vi "start_photon_stream.vi"(8 "error in (no error)":errorcluster, 11 "tt20 in":refnum<class "tt20.lvclass">) -> (0 "error out":errorcluster, 3 "tt20 out":refnum<class "tt20.lvclass">)   [LabVIEW 2015, in "tt20.lvclass"]
uses:
  tt20.lvclass
  tt20.lvclass/tt20.ctl
  tt20_buffer_tdef.ctl
  C:/Users/MX-Microscope/Documents/LabVIEW Data/lvoop_campus_2018/Detector_Class/Swabian/time_tagger_vis/TTCSharp32.dll
  time_tagger_vis/TTCSharp32.dll
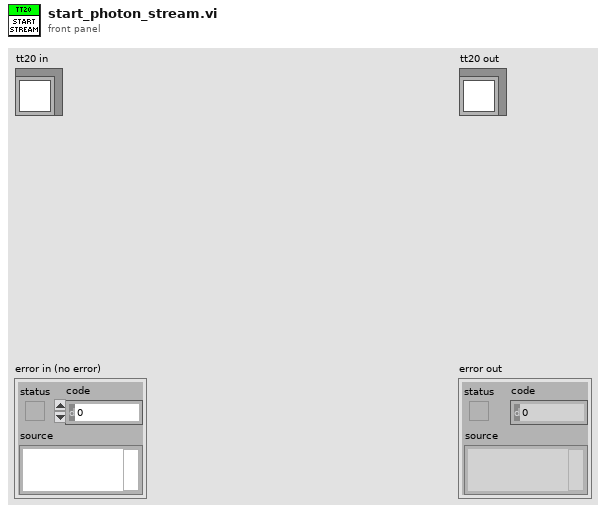
[diagram p1: front panel]
types:
  T1 = typedef "tt20_buffer_tdef.ctl" = cluster{"tagChannels":u32[], "tagTimestamps":i64[], "size":i32}
  T2 = typedef "tt20_acq_mode_tdef.ctl" = enum16{"T2", "T3"}
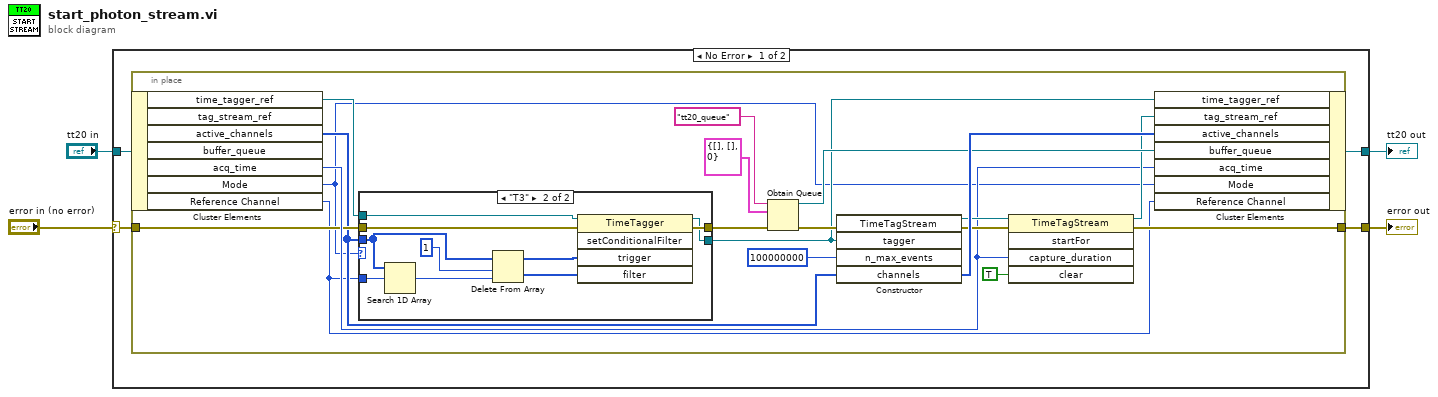
[diagram p0: block diagram]
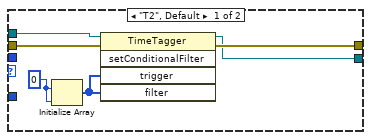
[diagram p2: hidden frame]
diagram:
  n1 = case shown="No Error" "error in (no error)" {
    selector: "error in (no error)" -> [w7 w44]
    tunnel: "tt20 in" -> [w8 w45]
    tunnel: [w6 w44] -> w2
    tunnel: [w5 w45] -> w1
    frame No Error {
      n2 = in-place {
        in-place-border: w7 -> [w15]
        in-place-border: [w19] -> w6
        n3 = in-place-cluster #1(w8) -> ("time_tagger_ref"=w13:refnum<k24>, "active_channels"=w11:u32[], "acq_time"=w16:i64, "Mode"=w10:T2, "Reference Channel"=w9:u8)  [unwired: 2 out]
        n4 = case shown="\"T3\"" w10 {
          tunnel: w15 -> [w33 w43]
          tunnel: [w32 w42] -> w14
          tunnel: w13 -> [w31 w41]
          tunnel: [w30 w40] -> w12
          tunnel: w11 -> [_ w38]
          tunnel: w9 -> [_ w39]
          frame "T2", Default {
            w29 = 0 ("dimension size")
            n5 = Initialize Array(w29, w29) -> (w28:i32[])
            n6 = invoke class="TimeTagger" method="setConditionalFilter"(reference=w31, error in=w33, "trigger"=w28, "filter"=w28) -> (reference out=w30:refnum<k24>, error out=w32:errorcluster)  [unwired: 1 in, 3 out]
          }
          frame "T3" {
            n7 = Search 1D Array(1D array=w38, element=w39) -> (index of element=w37:i32)  [unwired: 1 in]
            n8 = Delete From Array(array=w38, length=1, index=w37) -> (deleted portion=w34:u32[], array with subset deleted=w35:u32[])
            n9 = invoke class="TimeTagger" method="setConditionalFilter"(reference=w41, error in=w43, "trigger"=w35, "filter"=w34) -> (reference out=w40:refnum<k24>, error out=w42:errorcluster)  [unwired: 1 in, 3 out]
          }
        }
        n10 = Obtain Queue(name (unnamed)="tt20_queue", element data type=T1 {"tagChannels"=[], "tagTimestamps"=[], "size"=0} ("output cluster"), error in (no error)=w14) -> (queue out=w22:refnum<queue>, error out=w24:errorcluster)  [unwired: 2 in, 1 out]
        n11 = constructor class="TimeTagStream"(error in=w24, "tagger"=w12, "n_max_events"=100000000, "channels"=w11) -> (reference out=w21:refnum<k24>, error out=w17:errorcluster, "channels"=w26:u32[])  [unwired: 2 in, 3 out]
        n12 = invoke class="TimeTagStream" method="startFor"(reference=w21, error in=w17, "capture_duration"=w16, "clear"=TRUE) -> (reference out=w20:refnum<k24>, error out=w19:errorcluster)  [unwired: 1 in, 3 out]
        n13 = in-place-cluster #1("time_tagger_ref"=w12, "tag_stream_ref"=w20, "active_channels"=w26, "buffer_queue"=w22, "acq_time"=w16, "Mode"=w10, "Reference Channel"=w9) -> (w5:refnum<class "tt20.lvclass">)
      }
    }
    frame Error {
    }
  }
  "error out" <- w2
  "tt20 out" <- w1
